vi "Set Pot Zero.vi"(11 "Run?":bool) -> (3 "Run Again?":bool)   [LabVIEW 2014]
uses:
  <vilib>/Rock Robotics/WPI/Solenoid/Deprecated/WPI_SolenoidSetBool.vi
  Robot Global Data.vi
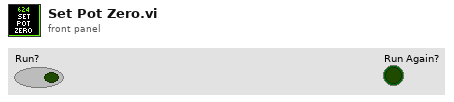
[diagram p1: front panel]
types:
  T1 = typedef "WPI_DriverStationRobotMode2.ctl" = enum16{"Autonomous Disabled", "Autonomous Enabled", "Teleop Disabled", "Teleop Enabled", "Disconnected", "Finish", "Test Disabled", "Test Enabled", "Emergency Stopped"}
  T2 = typedef "WPI_SolenoidDevRef.ctl" = cluster{"DevStatus":errorcluster, "Pneumatics Control Module":u8, "Forward Solenoid Channel":T3, "Reverse Solenoid Channel":T3}
  T3 = typedef "WPI_SolenoidChannel.ctl" = enum8{"Solenoid 0", "Solenoid 1", "Solenoid 2", "Solenoid 3", "Solenoid 4", "Solenoid 5", "Solenoid 6", "Solenoid 7", "Invalid"}
  T4 = typedef "WPI_PotentiometerDevRef.ctl" = cluster{"DevStatus":errorcluster, "Controller":T5, "Analog Channel":T6, "Invert Output":bool}
  T5 = typedef "FPGA_TypedefAnalogModule.ctl" = enum16{"Controller 1"}
  T6 = typedef "FPGA_AIChannel.ctl" = enum8{"AI 0", "AI 1", "AI 2", "AI 3", "AI MXP 0", "AI MXP 1", "AI MXP 2", "AI MXP 3", "Invalid"}
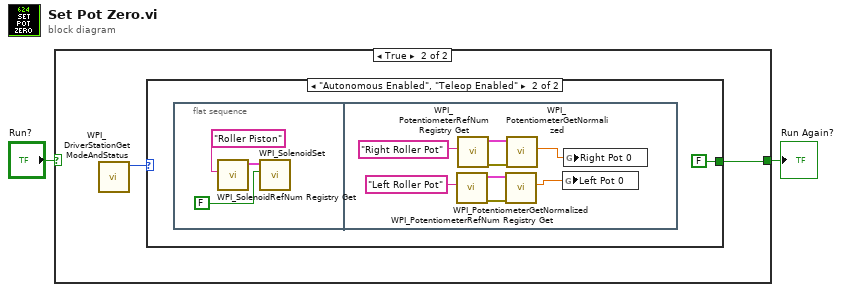
[diagram p0: block diagram]
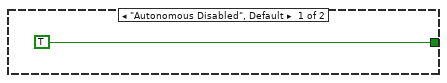
[diagram p3: hidden frame]
diagram:
  n1 = case shown="True" "Run?" {
    selector: "Run?" -> [w3 _]
    tunnel: [w3 w4] -> w1
    frame False {
    }
    frame True {
      n2 = call <vilib>:"WPI_DriverStationGetModeAndStatus.vi"() -> ("Robot Mode"=w5:T1)  [unwired: 10 in, 1 out]
      n3 = case shown="\"Autonomous Enabled\", \"Teleop Enabled\"" w5 {
        tunnel: [TRUE FALSE] -> w4
        frame "Autonomous Disabled", Default {
        }
        frame "Autonomous Enabled", "Teleop Enabled" {
          n4 = flat-sequence {
            frame #0 {
              n5 = call <vilib>:"WPI_SolenoidRefNum Registry Get.vi"("refnum name"="Roller Piston") -> ("SolenoidDevRef"=w10:T2)  [unwired: 9 in, 1 out]
              n6 = call-poly <vilib>:"WPI_SolenoidSet.vi"("Value"=FALSE, "SolenoidDevRef"=w10) -> ()  [unwired: 8 in, 2 out]
            }
            frame #1 {
              n7 = call <vilib>:"WPI_PotentiometerRefNum Registry Get.vi"("refnum name"="Left Roller Pot") -> ("error out"=w15:errorcluster, "PotDevRef"=w16:T4)  [unwired: 9 in]
              n8 = call <vilib>:"WPI_PotentiometerRefNum Registry Get.vi"("refnum name"="Right Roller Pot") -> ("error out"=w18:errorcluster, "PotDevRef"=w17:T4)  [unwired: 9 in]
              n9 = call <vilib>:"WPI_PotentiometerGetNormalized.vi"("error in"=w15, "PotDevRef"=w16) -> ("Normalized Value"=w12:dbl)  [unwired: 7 in, 2 out]
              n10 = call <vilib>:"WPI_PotentiometerGetNormalized.vi"("error in"=w18, "PotDevRef"=w17) -> ("Normalized Value"=w11:dbl)  [unwired: 7 in, 2 out]
              n11 = global write "Robot Global Data.vi" "Left Pot 0"(w12) -> ()
              n12 = global write "Robot Global Data.vi" "Right Pot 0"(w11) -> ()
            }
          }
        }
      }
    }
  }
  "Run Again?" <- w1
